vi "Write Data Refnum.vi"(8 "error in (no error)":errorcluster, 10 "Data Refnum":refnum<vi>, 11 "Display Panel Non-Actor Class in":refnum<class "Display Panel Non-Actor Class.lvclass">) -> (0 "error out":errorcluster, 3 "Display Panel Non-Actor Class out":refnum<class "Display Panel Non-Actor Class.lvclass">)   [LabVIEW 2013, in "Display Panel Non-Actor Class.lvlib" / "Display Panel Non-Actor Class.lvclass"]
uses:
  Display Panel Non-Actor Class.lvclass
  Controls/Numeric Indicator.ctl
  Display Panel Non-Actor Class.lvclass/Display Panel Non-Actor Class.ctl
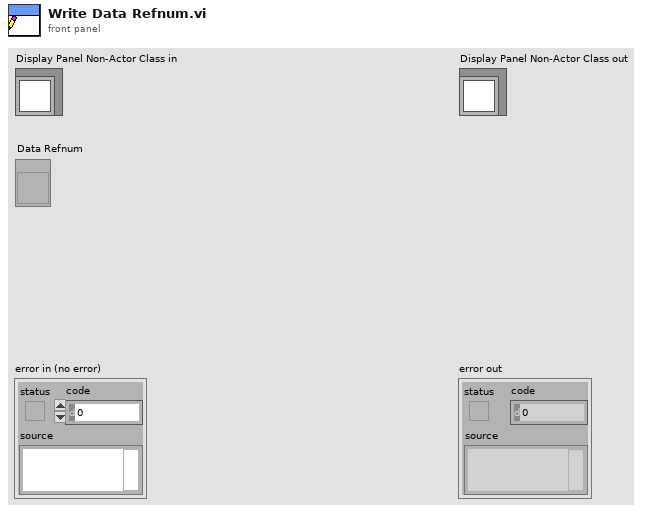
[diagram p1: front panel]
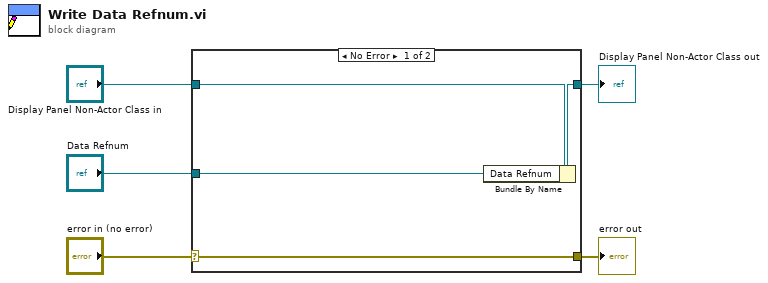
[diagram p0: block diagram]
diagram:
  n1 = case shown="No Error" "error in (no error)" {
    selector: "error in (no error)" -> [w9 w10]
    tunnel: [w9 w10] -> w4
    tunnel: [w7 w11] -> w2
    tunnel: "Display Panel Non-Actor Class in" -> [w8 w11]
    tunnel: "Data Refnum" -> [w6 _]
    frame No Error {
      n2 = Bundle By Name(cluster=w8, "Data Refnum"=w6) -> (w7:refnum<class "Display Panel Non-Actor Class.lvclass">)
    }
    frame Error {
    }
  }
  "error out" <- w4
  "Display Panel Non-Actor Class out" <- w2
